vi "Instantiate.vi"(1 "vi ref":refnum<vi>) -> (0 "vi ref":refnum<vi>)   [LabVIEW 2019, in "MessengerM.lvlib"]
doc: "Creates and initializes the data structure that supports the channel at run time."
uses:
  MessengerM.lvlib
  MessengerMBase/MessengerMBase.lvclass
  ChannelOp.ctl
  MessengerMCPU/MessengerMCPU.lvclass
  C:/Users/jimkring/Desktop/MessengerM/MultiStation Controller/MessengerM/MessengerMBase/MessengerMBase.lvclass
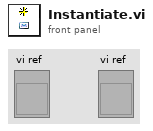
[diagram p1: front panel]
types:
  T1 = typedef "MessengerM.lvlib/ChannelOp.ctl" = enum16{"init", "write", "read", "wrtAck", "rdAck", "rdAck2", "probe"}
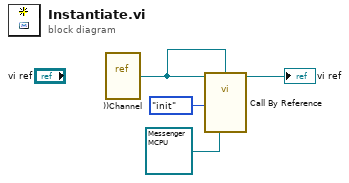
[diagram p0: block diagram]
diagram:
  n1 = vi-ref "))Channel.vi"() -> (w4:refnum<vi>)
  n2 = call-by-ref "?"(reference=w4, "This VI"=w4, "channelOp"=ChannelOp."init", "replacement"=refnum<class "MessengerMCPU.lvclass"> refnum ("Messenger:MessengerMCPU.lvclass")) -> (reference out=→"vi ref":refnum<vi>)  [unwired: 9 in, 6 out]
